vi "Stop Driving.vi"(7 "Description":string, 8 "Command Info In":T1) -> (0 "Command Info Out":T1)   [LabVIEW 2020]
doc: "Zero the drive motors, making the robot stationary."
uses:
  <vilib>/Rock Robotics/WPI/Framework/Command Status Info.ctl
  <vilib>/Rock Robotics/WPI/Framework/Completion Status.ctl
  <vilib>/Rock Robotics/WPI/Framework/Completion Notifier.ctl
  Implementation/Drive Setpoints.ctl
  Implementation/Drive Operations.ctl
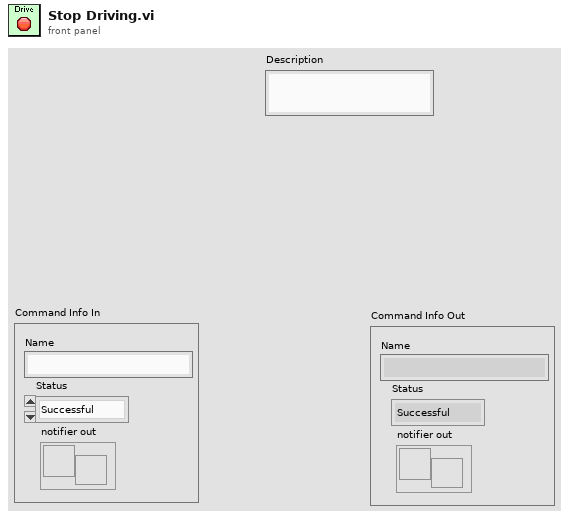
[diagram p1: front panel]
types:
  T1 = typedef "Command Status Info.ctl" = cluster{"Name":string, "Status":T2, "notifier out":T3}
  T2 = typedef "Completion Status.ctl" = enum16{"Successful", "Aborted", "Incomplete"}
  T3 = typedef "Completion Notifier.ctl" = refnum<notifier>
  T4 = typedef "Drive Setpoints.ctl" = cluster{"Operation":T5, "Left Setpoint":dbl, "Right Setpoint":dbl, "Duration":dbl}
  T5 = typedef "Drive Operations.ctl" = enum16{"Reserve", "Read Current", "Immediate", "Drive for Time", "Drive for Distance", "Stop Driving"}
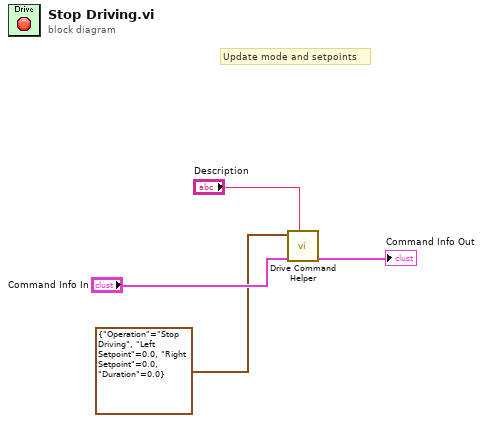
[diagram p0: block diagram]
diagram:
  # "Update mode and setpoints"
  n1 = call "Drive Command Helper.vi"("Description"="Description", "Command Info In"="Command Info In", "SubSystem Data"=T4 {"Operation"=enum."Stop Driving", "Left Setpoint"=0.0, "Right Setpoint"=0.0, "Duration"=0.0}) -> ("Command Info Out"=→"Command Info Out":T1)  [unwired: 6 in, 2 out]
